vi "SDT_ReadMeasureInfoBlock.vi"(8 "error in":errorcluster, 10 "bhfile_header":T11 {"chksum" format="x%x"; "header_valid" format="x%x"}, 11 "SDTFileRefnum":refnum<file>) -> (0 "error out":errorcluster, 1 "MeasureInfo":T1[](array[typedef]) {"MeasFCSInfo"."fcs_decay_calc" format="%x"; "MeasStopInfo"."flags" format="x%x"; "MeasureInfo_PartB"."mod_type2" format="%016x"; "MeasureInfo_PartB"."mod_type1" format="%016x"}, 3 "SDTFileRefnum":refnum<file>)   [LabVIEW 2019]
doc: "This VI is a SubVI to SDT_ReadFile.vi. It reads the MeasureInfo block in a SDT-file from disc.\nFor a description of the *.sdt file format see: SPC_data_file_structure.h\n\ninfo@becker-hickl.com"
uses:
  SPC_Controls/bhfile_header.ctl
  SPC_Controls/MeasureInfo.ctl
  SPC_Controls/MeasureInfo_PartB.ctl
  SPC_Controls/MeasStopInfo.ctl
  SPC_Controls/MeasFCSInfo.ctl
  SPC_Controls/MeasureInfo_PartE.ctl
  SPC_Controls/MeasHISTInfo.ctl
  SPC_Controls/HISTInfoExt.ctl
  SPC_Controls/MeasureInfo_PartI.ctl
  SPC_Controls/MeasureInfo_PartK.ctl
  SPC_Controls/MeasureInfo_PartM.ctl
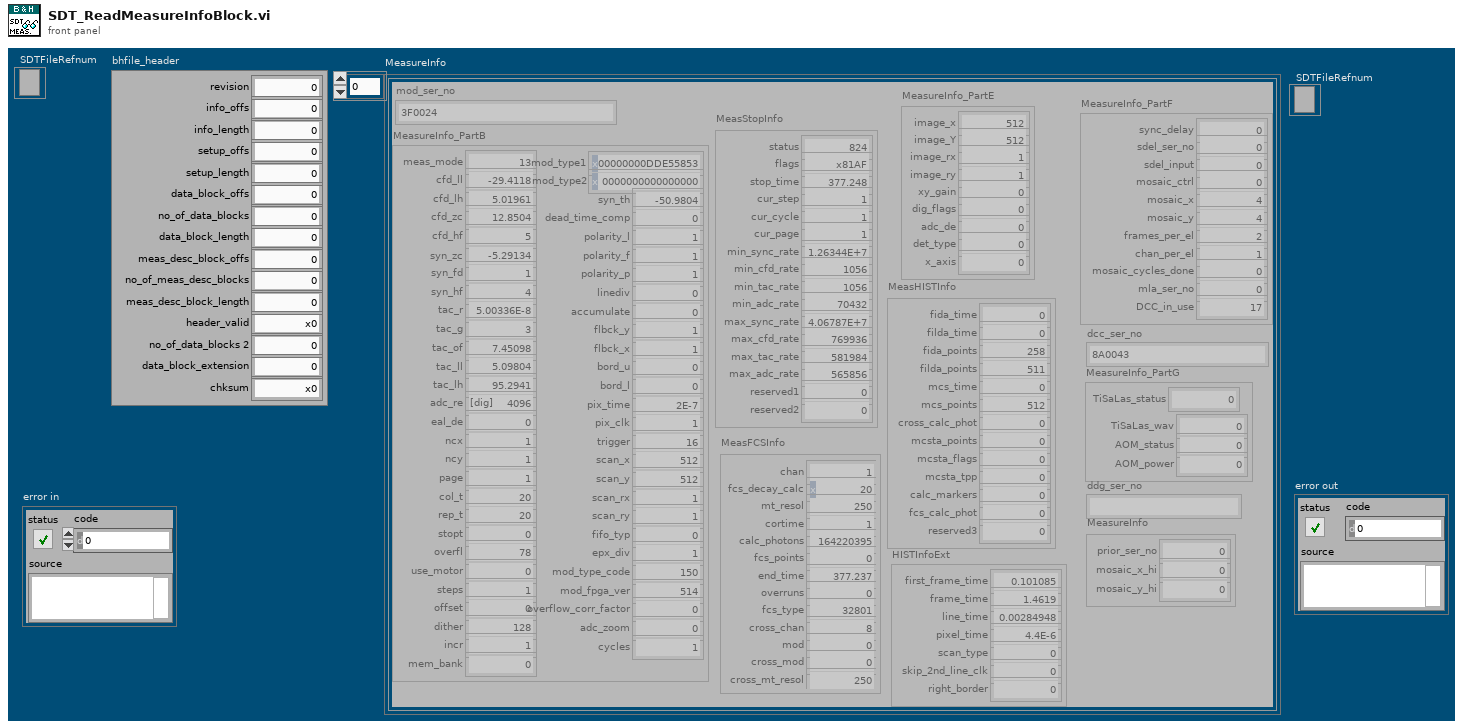
[diagram p1: front panel]
types:
  T1 = typedef "MeasureInfo.ctl" = cluster{"mod_ser_no":string, "MeasureInfo_PartB":T2, "MeasStopInfo":T3, "MeasFCSInfo":T4, "MeasureInfo_PartE":T5, "MeasHISTInfo":T6, "HISTInfoExt":T7, "MeasureInfo_PartF":T8, "dcc_ser_no":string, "MeasureInfo_PartG":T9, "ddg_ser_no":string, "MeasureInfo":T10}
  T2 = typedef "MeasureInfo_PartB.ctl" = cluster{"meas_mode":i16, "cfd_ll":sgl, "cfd_lh":sgl, "cfd_zc":sgl, "cfd_hf":sgl, "syn_zc":sgl, "syn_fd":i16, "syn_hf":sgl, "tac_r":sgl, "tac_g":i16, "tac_of":sgl, "tac_ll":sgl, "tac_lh":sgl, "adc_re":i16, "eal_de":i16, "ncx":i16, "ncy":i16, "page":u16, "col_t":sgl, "rep_t":sgl, "stopt":i16, "overfl":i8, "use_motor":i16, "steps":u16, "offset":sgl, "dither":i16, "incr":i16, "mem_bank":i16, "mod_type1":u64, "mod_type2":u64, "syn_th":sgl, "dead_time_comp":i16, "polarity_l":i16, "polarity_f":i16, "polarity_p":i16, "linediv":i16, "accumulate":i16, "flbck_y":i32, "flbck_x":i32, "bord_u":i32, "bord_l":i32, "pix_time":sgl, "pix_clk":i16, "trigger":i16, "scan_x":i32, "scan_y":i32, "scan_rx":i32, "scan_ry":i32, "fifo_typ":i16, "epx_div":i32, "mod_type_code":u16, "mod_fpga_ver":u16, "overflow_corr_factor":sgl, "adc_zoom":i32, "cycles":i32}
  T3 = typedef "MeasStopInfo.ctl" = cluster{"status":u16, "flags":u16, "stop_time":sgl, "cur_step":i32, "cur_cycle":i32, "cur_page":i32, "min_sync_rate":sgl, "min_cfd_rate":sgl, "min_tac_rate":sgl, "min_adc_rate":sgl, "max_sync_rate":sgl, "max_cfd_rate":sgl, "max_tac_rate":sgl, "max_adc_rate":sgl, "reserved1":i32, "reserved2":sgl}
  T4 = typedef "MeasFCSInfo.ctl" = cluster{"chan":u16, "fcs_decay_calc":u16, "mt_resol":u32, "cortime":sgl, "calc_photons":u32, "fcs_points":i32, "end_time":sgl, "overruns":u16, "fcs_type":u16, "cross_chan":u16, "mod":u16, "cross_mod":u16, "cross_mt_resol":u32}
  T5 = typedef "MeasureInfo_PartE.ctl" = cluster{"image_x":i32, "image_Y":i32, "image_rx":i32, "image_ry":i32, "xy_gain":i16, "dig_flags":i16, "adc_de":i16, "det_type":i16, "x_axis":i16}
  T6 = typedef "MeasHISTInfo.ctl" = cluster{"fida_time":sgl, "filda_time":sgl, "fida_points":i32, "filda_points":i32, "mcs_time":sgl, "mcs_points":i32, "cross_calc_phot":u32, "mcsta_points":u16, "mcsta_flags":u16, "mcsta_tpp":u32, "calc_markers":u32, "fcs_calc_phot":u32, "reserved3":u32}
  T7 = typedef "HISTInfoExt.ctl" = cluster{"first_frame_time":sgl, "frame_time":sgl, "line_time":sgl, "pixel_time":sgl, "scan_type":i16, "skip_2nd_line_clk":i16, "right_border":u32}
  T8 = typedef "MeasureInfo_PartI.ctl" = cluster{"sync_delay":sgl, "sdel_ser_no":u16, "sdel_input":i8, "mosaic_ctrl":i8, "mosaic_x":u8, "mosaic_y":u8, "frames_per_el":i16, "chan_per_el":i16, "mosaic_cycles_done":i32, "mla_ser_no":u16, "DCC_in_use":u8}
  T9 = typedef "MeasureInfo_PartK.ctl" = cluster{"TiSaLas_status":u16, "TiSaLas_wav":u16, "AOM_status":u8, "AOM_power":u8}
  T10 = typedef "MeasureInfo_PartM.ctl" = cluster{"prior_ser_no":i32, "mosaic_x_hi":u8, "mosaic_y_hi":u8}
  T11 = typedef "bhfile_header.ctl" = cluster{"revision":i16, "info_offs":i32, "info_length":i16, "setup_offs":i32, "setup_length":u16, "data_block_offs":i32, "no_of_data_blocks":i16, "data_block_length":u32, "meas_desc_block_offs":i32, "no_of_meas_desc_blocks":i16, "meas_desc_block_length":i16, "header_valid":u16, "no_of_data_blocks 2":u32, "data_block_extension":u16, "chksum":u16}
  T12 = enum16{"big-endian, network order", "native, host order", "little-endian"}
  T13 = cluster{string, "MeasureInfo_PartB":T2, "MeasStopInfo":T3, "MeasFCSInfo":T4, "MeasureInfo_PartE":T5, "MeasHISTInfo":T6, "HISTInfoExt":T7, "MeasureInfo_PartF":T8, string, "MeasureInfo_PartG":T9, string, "MeasureInfo":T10}
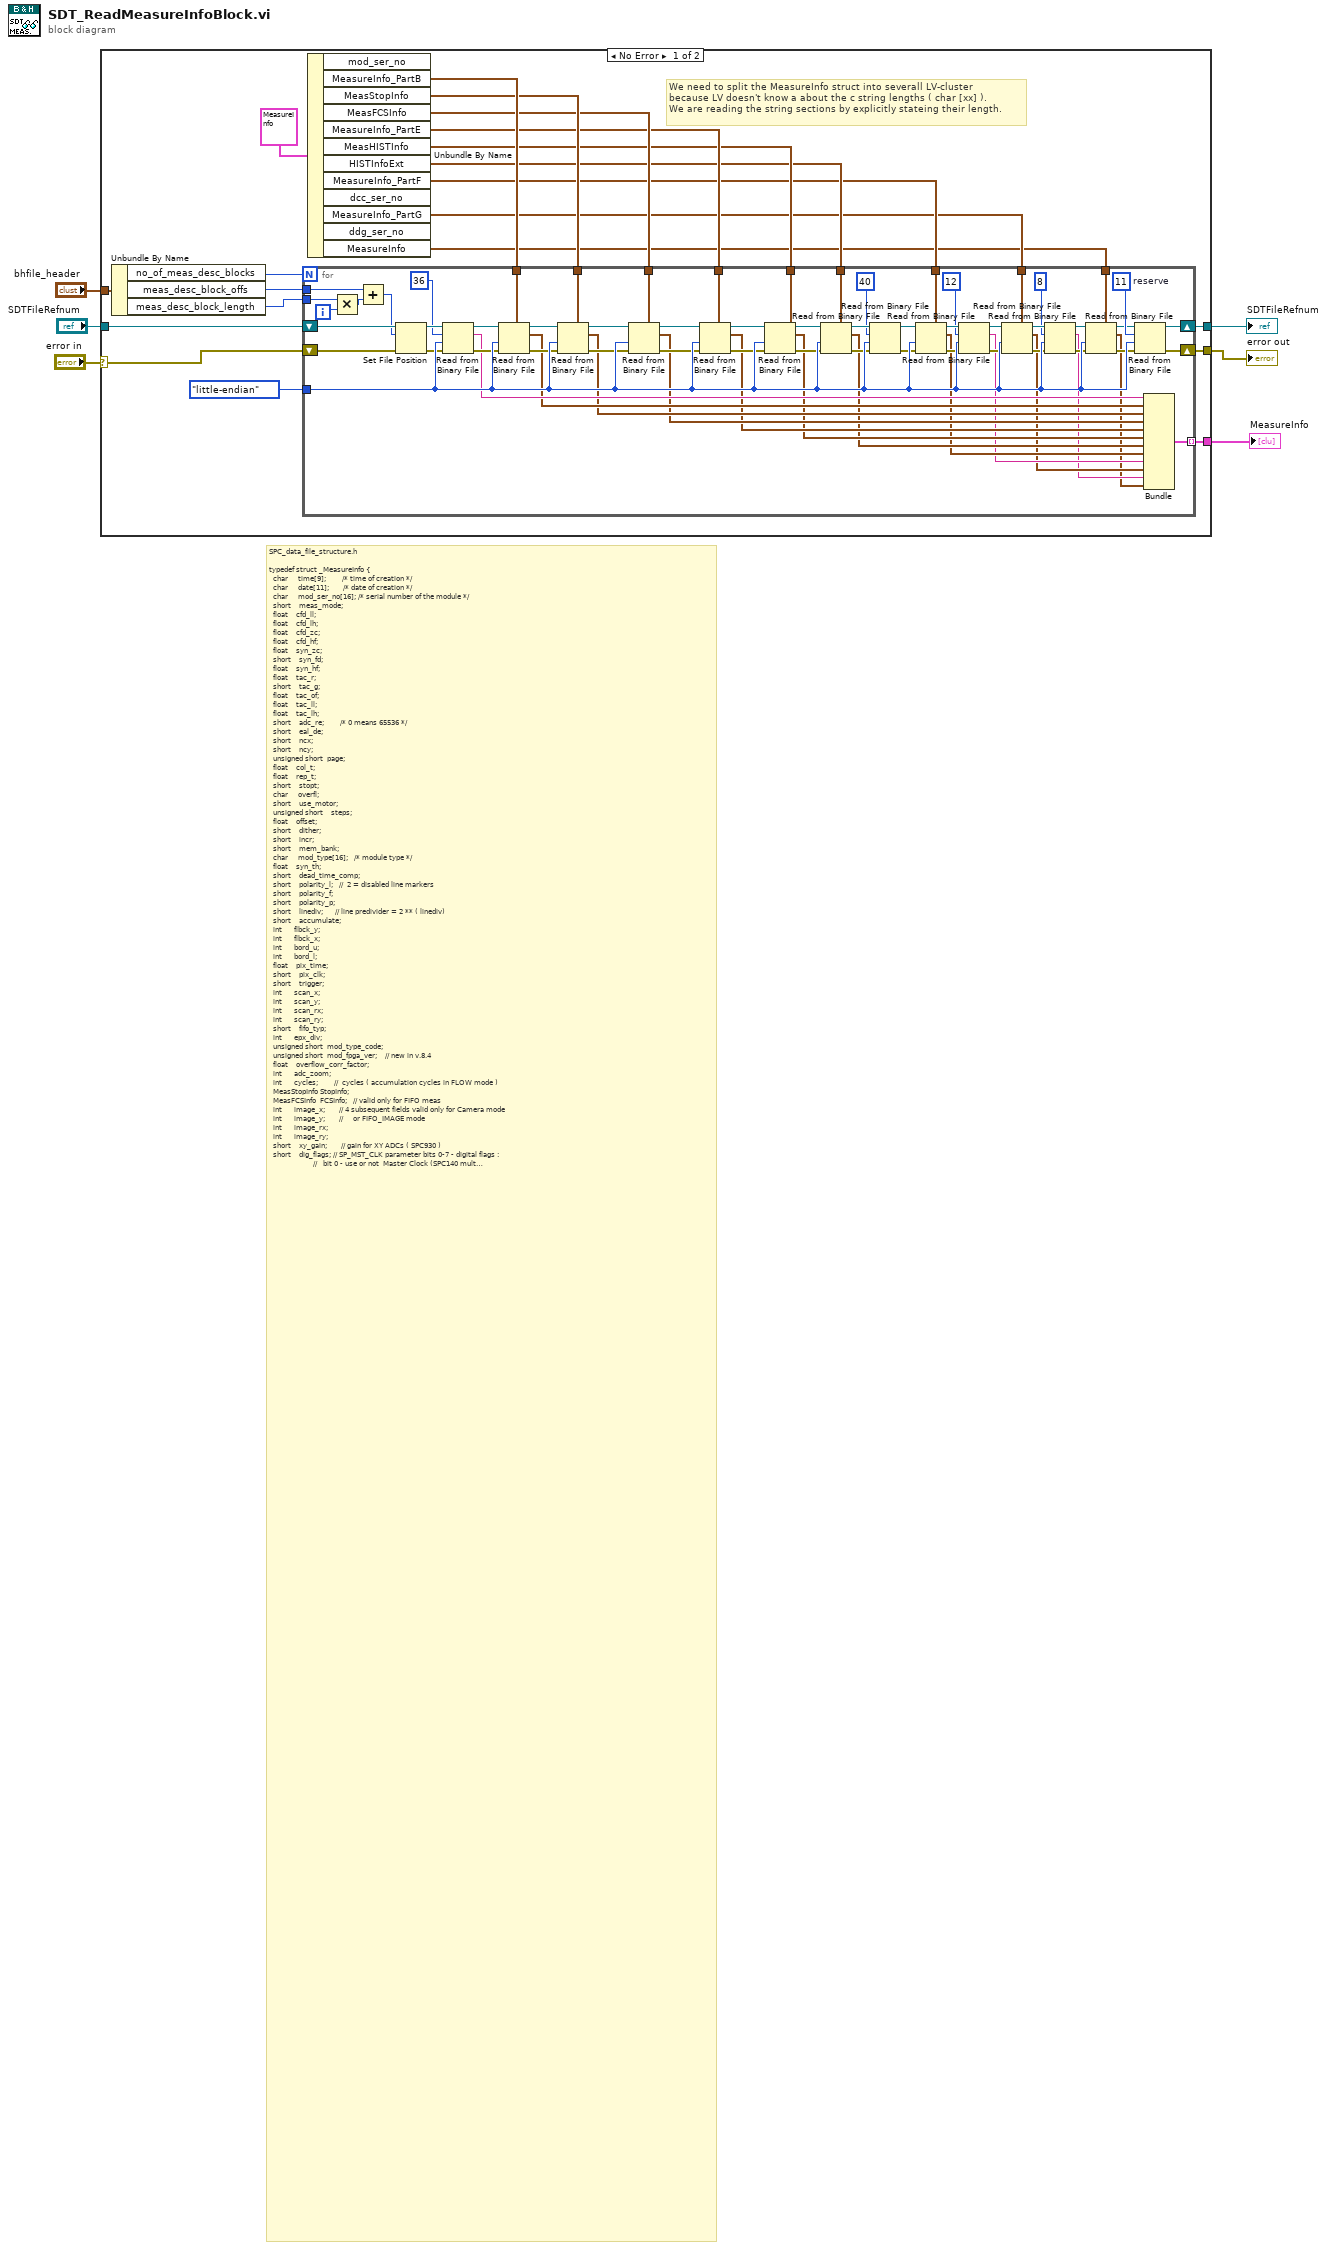
[diagram p0: block diagram]
diagram:
  # "SPC_data_file_structure.h\n\ntypedef struct _MeasureInfo {\n  char     time[9];        /* time of creation */\n  char     date[11];       /* date of creation */\n  char     mod_ser_no[16]; /* serial number of the module */\n  short    meas_mode;\n  float    cfd_ll;\n  float    cfd_lh;\n  float    cfd_zc;\n  float    cfd_hf;\n  float    syn_zc;\n  short    syn_fd;\n  float    syn_hf;\n  float    tac_r;\n  short    tac_g;\n  float    tac_of;\n  float    tac_ll;\n  float    tac_lh;\n  short    adc_re;        /* 0 means 65536 */\n  short    eal_de;\n  short    ncx;\n  short    ncy;\n  unsigned short  page;\n  float    col_t;\n  float    rep_t;\n  short    stopt;\n  char     overfl;\n  short    use_motor;\n  unsigned short    steps;\n  float    offset;\n  short    dither;\n  short    incr;\n  short    mem_bank;\n  char     mod_type[16];   /* module type */\n  float    syn_th;\n  short    dead_time_comp;\n  short    polarity_l;   //  2 = disabled line markers\n  short    polarity_f;\n  short    polarity_p;\n  short    linediv;      // line predivider = 2 ** ( linediv)\n  short    accumulate;\n  int      flbck_y; \n  int      flbck_x; \n  int      bord_u; \n  int      bord_l; \n  float    pix_time;\n  short    pix_clk; \n  short    trigger; \n  int      scan_x; \n  int      scan_y; \n  int      scan_rx; \n  int      scan_ry; \n  short    fifo_typ;\n  int      epx_div; \n  unsigned short  mod_type_code; \n  unsigned short  mod_fpga_ver;    // new in v.8.4\n  float    overflow_corr_factor;\n  int      adc_zoom; \n  int      cycles;        //  cycles ( accumulation cycles in FLOW mode ) \n  MeasStopInfo StopInfo;\n  MeasFCSInfo  FCSInfo;   // valid only for FIFO meas\n  int      image_x;       // 4 subsequent fields valid only for Camera mode\n  int      image_y;       //     or FIFO_IMAGE mode\n  int      image_rx; \n  int      image_ry; \n  short    xy_gain;       // gain for XY ADCs ( SPC930 )\n  short    dig_flags; // SP_MST_CLK parameter bits 0-7 - digital flags : \n                      //   bit 0 - use or not  Master Clock (SPC140 multi-module )\n                      //   bit 1 - Continuous Flow On/Off for scan modes in SPC150\n                      //   bit 2 - time(X) axis of decay curves reversed by software(1), or not (0)\n  short    adc_de;        // ADC sample delay ( SPC-930 )\n  short    det_type;      // detector type ( SPC-930 in camera mode ) \n  short    x_axis;        // X axis representation ( SPC-930 ) \n  MeasHISTInfo  HISTInfo; // extension of FCSInfo, valid only for FIFO meas\n  MeasHISTInfoExt  HISTInfoExt; // extension of HSTInfo, valid only for FIFO meas\n  float    sync_delay;    // Sync Delay [ns] when using BH SyncDel USB box\n  unsigned short sdel_ser_no;  // serial number of Sync Delay box, \n                               //         = 0 - SyncDelay box was not used  \n  char     sdel_input;    // active input of SyncDelay box, 0 - IN 1, 1 - IN 2                         \n  char     mosaic_ctrl;   // bit 0 - mosaic imaging was used, \n                          // bit 1 - mosaic type ( 000 - sequence of frames, 001 - rout. channels)\n                          // bit 2-3 - mosaic restart type ( 0 - no, 1 - Marker 3, 2 - Ext. trigger\n                          // bit 4-5 - mosaic type extension( \n                          //               010 - sequence of Z planes of Axio Observer.Z1)\n                          //               011 - sequence of frames with motor stage )\n  unsigned char     mosaic_x;      //  no of mosaic elements in X dir.  (lower 8 bits )\n  unsigned char     mosaic_y;      //  no of mosaic elements in Y dir.  (lower 8 bits )\n  short    frames_per_el; //  frames per mosaic element 1 .. 32767\n  short    chan_per_el;   //  routing channels per mosaic element 1 .. 256\n  int      mosaic_cycles_done;  // number of mosaic accumulation cycles done \n  unsigned short mla_ser_no;  // serial number of MLA4 device, \n                               //         = 0 - MLA4 device was not used \n  unsigned char  DCC_in_use;  // bits 0..3 = 1 when DCC module M1..M4 was in use\n  char     dcc_ser_no[12];    //  serial number of used DCC module\n  unsigned short TiSaLas_status;  //  laser status :bit 0 - used or not, b1 - present,\n                   // b2 - on/off, b3 - shutter, b4 - warm up, b5 - pulsing, \n                   // b6 - error, b7-10 - laser type 0-15, 0 = unknown \n  unsigned short TiSaLas_wav;  //  laser wavelength in nm\n  unsigned char  AOM_status;   //  AOM status :bit 0 - used or not, b1 - present,\n                               //              b2 - modulation, b3 - remote, b4 - error\n  unsigned char  AOM_power;    //  AOM power in %  0 - 100 \n  char     ddg_ser_no[8];    //  serial number of used DDG module,\n                              //         = 0 - DDG module was not used \n  int      prior_ser_no;      // serial number of used Prior device, 0 - not used\n  unsigned char     mosaic_x_hi;      //  no of mosaic elements in X dir.  (higher 8 bits )\n  unsigned char     mosaic_y_hi;      //  no of mosaic elements in Y dir.  (higher 8 bits )\n  char     reserve[11];       // total size of old MeasureInfo = 512 bytes\n  char     extension_used;    // MeasureInfoExt used\n  MeasureInfoExt  minfo_ext;  // extension structure - size fixed to 1536 bytes \n                              // new total size of MeasureInfo = 2048 bytes\n  }MeasureInfo;"
  n1 = case shown="No Error" "error in" {
    selector: "error in" -> [w8 w92]
    tunnel: "bhfile_header" -> [w24 _]
    tunnel: "SDTFileRefnum" -> [w22 w93]
    tunnel: [w21 _] -> w4
    tunnel: [w10 w93] -> w3
    tunnel: [w7 w92] -> w1
    frame No Error {
      # "We need to split the MeasureInfo struct into severall LV-cluster\nbecause LV doesn't know a about the c string lengths ( char [xx] ).\nWe are reading the string sections by explicitly stateing their length."
      n2 = Unbundle By Name(w24) -> ("no_of_meas_desc_blocks"=w25:i16, "meas_desc_block_offs"=w26:i32, "meas_desc_block_length"=w9:i16)
      n3 = Unbundle By Name(T1 {"mod_ser_no"="3F0024\u0000\u0000\u0000\u0000\u0000\u0000\u0000\u0000\u0000\u0000", "MeasureInfo_PartB"={"meas_mode"=13, "cfd_ll"=-29.411764, "cfd_lh"=5.019608, "cfd_zc"=12.850393, "cfd_hf"=5.0, "syn_zc"=-5.2913384, "syn_fd"=1, "syn_hf"=4.0, "tac_r"=5.0033574e-08, "tac_g"=3, "tac_of"=7.45098, "tac_ll"=5.098039, "tac_lh"=95.29412, "adc_re"=4096, "eal_de"=0, "ncx"=1, "ncy"=1, "page"=1, "col_t"=20.0, "rep_t"=20.0, "stopt"=0, "overfl"=78, "use_motor"=0, "steps"=1, "offset"=0.0, "dither"=128, "incr"=1, "mem_bank"=0, "mod_type1"=3722795091, "mod_type2"=0, "syn_th"=-50.980392, "dead_time_comp"=0, "polarity_l"=1, "polarity_f"=1, "polarity_p"=1, "linediv"=0, "accumulate"=0, "flbck_y"=1, "flbck_x"=1, "bord_u"=0, "bord_l"=0, "pix_time"=2e-07, "pix_clk"=1, "trigger"=16, "scan_x"=512, "scan_y"=512, "scan_rx"=1, "scan_ry"=1, "fifo_typ"=0, "epx_div"=1, "mod_type_code"=150, "mod_fpga_ver"=514, "overflow_corr_factor"=0.0, "adc_zoom"=0, "cycles"=1}, "MeasStopInfo"={"status"=824, "flags"=33199, "stop_time"=377.24805, "cur_step"=1, "cur_cycle"=1, "cur_page"=1, "min_sync_rate"=12634368.0, "min_cfd_rate"=1056.0, "min_tac_rate"=1056.0, "min_adc_rate"=70432.0, "max_sync_rate"=40678656.0, "max_cfd_rate"=769936.0, "max_tac_rate"=581984.0, "max_adc_rate"=565856.0, "reserved1"=0, "reserved2"=0.0}, "MeasFCSInfo"={"chan"=1, "fcs_decay_calc"=32, "mt_resol"=250, "cortime"=1.0, "calc_photons"=164220395, "fcs_points"=0, "end_time"=377.2369, "overruns"=0, "fcs_type"=32801, "cross_chan"=8, "mod"=0, "cross_mod"=0, "cross_mt_resol"=250}, "MeasureInfo_PartE"={"image_x"=512, "image_Y"=512, "image_rx"=1, "image_ry"=1, "xy_gain"=0, "dig_flags"=0, "adc_de"=0, "det_type"=0, "x_axis"=0}, "MeasHISTInfo"={"fida_time"=0.0, "filda_time"=0.0, "fida_points"=258, "filda_points"=511, "mcs_time"=0.0, "mcs_points"=512, "cross_calc_phot"=0, "mcsta_points"=0, "mcsta_flags"=0, "mcsta_tpp"=0, "calc_markers"=0, "fcs_calc_phot"=0, "reserved3"=0}, "HISTInfoExt"={"first_frame_time"=0.10108537, "frame_time"=1.4619007, "line_time"=0.002849475, "pixel_time"=4.4e-06, "scan_type"=0, "skip_2nd_line_clk"=0, "right_border"=0}, "MeasureInfo_PartF"={"sync_delay"=0.0, "sdel_ser_no"=0, "sdel_input"=0, "mosaic_ctrl"=0, "mosaic_x"=4, "mosaic_y"=4, "frames_per_el"=2, "chan_per_el"=1, "mosaic_cycles_done"=0, "mla_ser_no"=0, "DCC_in_use"=17}, "dcc_ser_no"="8A0043\u0000\u0000\u0000\u0000\u0000\u0000", "MeasureInfo_PartG"={"TiSaLas_status"=0, "TiSaLas_wav"=0, "AOM_status"=0, "AOM_power"=0}, "ddg_ser_no"="\u0000\u0000\u0000\u0000\u0000\u0000\u0000\u0000", "MeasureInfo"={"prior_ser_no"=0, "mosaic_x_hi"=0, "mosaic_y_hi"=0}} ("MeasureInfo")) -> ("MeasureInfo_PartB"=w19:T2, "MeasStopInfo"=w18:T3, "MeasFCSInfo"=w17:T4, "MeasureInfo_PartE"=w16:T5, "MeasHISTInfo"=w15:T6, "HISTInfoExt"=w14:T7, "MeasureInfo_PartF"=w13:T8, "MeasureInfo_PartG"=w12:T9, "MeasureInfo"=w11:T10)  [unwired: 3 out]
      n4 = for {
        N: w25 -> [_]
        tunnel: w26 -> [w90]
        tunnel: T12."little-endian" ("byte order (0:big-endian, network order)") -> [w57]
        shift-right: [w59] -> w10
        shift-left: w22 -> [w85]
        tunnel: w9 -> [w81]
        tunnel: w19 -> [w80]
        tunnel: w18 -> [w79]
        tunnel: w17 -> [w78]
        tunnel: w16 -> [w77]
        tunnel: w15 -> [w75]
        tunnel: w14 -> [w73]
        tunnel: w13 -> [w70]
        tunnel: w12 -> [w64]
        tunnel: w11 -> [w58]
        tunnel: [w55] -> w21 mode=indexing
        shift-right: [w40] -> w7
        shift-left: w8 -> [w39]
        i -> [w83]
        w62 = 11  # reserve
        n5 = Multiply(x=w81, y=w83) -> (x*y=w82:i32)
        n6 = Add(x=w90, y=w82) -> (x+y=w84:i32)
        n7 = Set File Position(offset (in bytes) (0)=w84, refnum=w85, error in=w39) -> (refnum out=w91:refnum<file>, error out=w54:errorcluster)  [unwired: 1 in]
        n8 = Read from Binary File(8:w54, 9:w57, 10:36 ("count (1)"), 11:w91) -> (0:w53:errorcluster, 2:w38:string, 3:w56:refnum<file>)  [unwired: 2 in, 1 out]
        n9 = Read from Binary File(5:w80, 8:w53, 9:w57, 11:w56) -> (0:w52:errorcluster, 2:w37:T2, 3:w88:refnum<file>)  [unwired: 2 in, 1 out]
        n10 = Read from Binary File(5:w79, 8:w52, 9:w57, 11:w88) -> (0:w51:errorcluster, 2:w36:T3, 3:w87:refnum<file>)  [unwired: 2 in, 1 out]
        n11 = Read from Binary File(5:w78, 8:w51, 9:w57, 11:w87) -> (0:w50:errorcluster, 2:w35:T4, 3:w86:refnum<file>)  [unwired: 2 in, 1 out]
        n12 = Read from Binary File(5:w77, 8:w50, 9:w57, 11:w86) -> (0:w49:errorcluster, 2:w34:T5, 3:w76:refnum<file>)  [unwired: 2 in, 1 out]
        n13 = Read from Binary File(5:w75, 8:w49, 9:w57, 11:w76) -> (0:w48:errorcluster, 2:w33:T6, 3:w74:refnum<file>)  [unwired: 2 in, 1 out]
        n14 = Read from Binary File(5:w73, 8:w48, 9:w57, 11:w74) -> (0:w47:errorcluster, 2:w32:T7, 3:w72:refnum<file>)  [unwired: 2 in, 1 out]
        n15 = Read from Binary File(8:w47, 9:w57, 10:40 ("count (1)"), 11:w72) -> (0:w46:errorcluster, 3:w69:refnum<file>)  [unwired: 2 in, 2 out]
        n16 = Read from Binary File(5:w70, 8:w46, 9:w57, 11:w69) -> (0:w45:errorcluster, 2:w31:T8, 3:w68:refnum<file>)  [unwired: 2 in, 1 out]
        n17 = Read from Binary File(8:w45, 9:w57, 10:12 ("count (1)"), 11:w68) -> (0:w44:errorcluster, 2:w30:string, 3:w65:refnum<file>)  [unwired: 2 in, 1 out]
        n18 = Read from Binary File(5:w64, 8:w44, 9:w57, 11:w65) -> (0:w43:errorcluster, 2:w29:T9, 3:w66:refnum<file>)  [unwired: 2 in, 1 out]
        n19 = Read from Binary File(8:w43, 9:w57, 10:8 ("count (1)"), 11:w66) -> (0:w42:errorcluster, 2:w28:string, 3:w60:refnum<file>)  [unwired: 2 in, 1 out]
        n20 = Read from Binary File(5:w58, 8:w42, 9:w57, 11:w60) -> (0:w41:errorcluster, 2:w27:T10, 3:w61:refnum<file>)  [unwired: 2 in, 1 out]
        n21 = Read from Binary File(8:w41, 9:w57, 10:w62, 11:w61) -> (0:w40:errorcluster, 3:w59:refnum<file>)  [unwired: 2 in, 2 out]
        n22 = Bundle(w38, "MeasureInfo_PartB"=w37, "MeasStopInfo"=w36, "MeasFCSInfo"=w35, "MeasureInfo_PartE"=w34, "MeasHISTInfo"=w33, "HISTInfoExt"=w32, "MeasureInfo_PartF"=w31, w30, "MeasureInfo_PartG"=w29, w28, "MeasureInfo"=w27) -> (w55:T13)  [unwired: 1 in]
      }
    }
    frame Error {
    }
  }
  "MeasureInfo" <- w4
  "SDTFileRefnum" <- w3
  "error out" <- w1
